vi "processData.vi"(8 "error in (no error)":errorcluster, 10 "model":refnum<class "Model.lvclass">, 11 "WaitingForSettledPState in":refnum<class "WaitingForSettledPState.lvclass">) -> (0 "error out":errorcluster, 2 "model 2":refnum<class "Model.lvclass">, 3 "WaitingForSettledPState out":refnum<class "WaitingForSettledPState.lvclass">)   [LabVIEW 2015, in "WaitingForSettledPState.lvclass"]
uses:
  WaitingForSettledPState.lvclass
  Model/Model/Model.lvclass
  PreconditioningState/PreconditioningState.lvclass
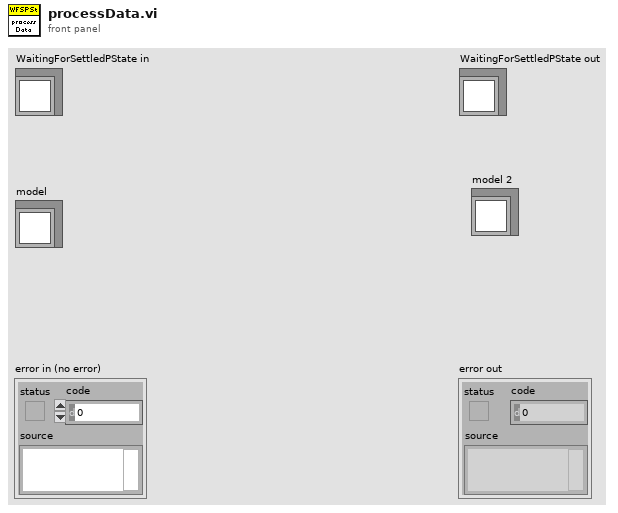
[diagram p1: front panel]
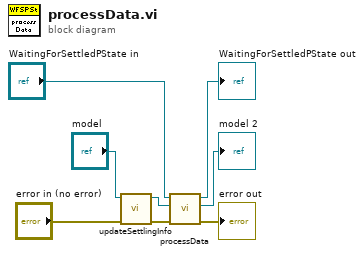
[diagram p0: block diagram]
diagram:
  n1 = call "updateSettlingInfo.vi"("error in (no error)"="error in (no error)", "Model in"="model") -> ("error out"=w3:errorcluster, "Model out"=w2:refnum<class "Model.lvclass">)  [unwired: 8 in]
  n2 = call-parent "processData.vi"("error in (no error)"=w3, "model"=w2, "TestingState in"="WaitingForSettledPState in") -> ("error out"=→"error out":errorcluster, "model 2"=→"model 2":refnum<class "Model.lvclass">, "TestingState out"=→"WaitingForSettledPState out":refnum<class "WaitingForSettledPState.lvclass">)  [unwired: 6 in]
